vi "Network Address Lookup Table.vi"(7 "Action":T3, 8 "error in (no error)":errorcluster, 9 "Address":u8, 10 "Data":T2 {"Name" format="%.0x"}, 11 "Address LUT":T1) -> (0 "error out":errorcluster {"code" min=0 max=0}, 1 "Found?":bool, 2 "Data":T2 {"Name" format="%.0x"}, 3 "Address LUT out":T1, 4 "All Data":T2[](array[typedef]) {"Name" format="%.0x"})   [LabVIEW 2015, in "J1939 Addon Engine.lvlib"]
uses:
  J1939 Addon Engine.lvlib
  J1939 Multi Packet Frame/Types/Address Table Reference.ctl
  Shared/Types/Address Lookup Table Data.ctl
  J1939 Multi Packet Frame/Types/Address Lookup Table Action.ctl
  Shared/J1939 Addon Shared.lvlib
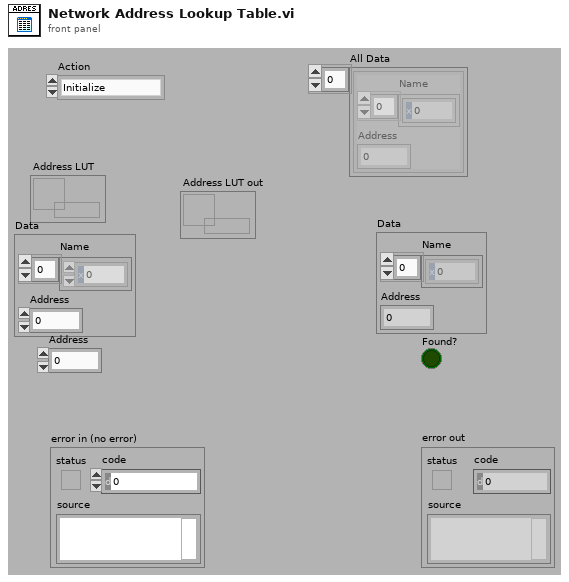
[diagram p1: front panel]
types:
  T1 = typedef "J1939 Addon Engine.lvlib/Address Table Reference.ctl" = refnum<data-value>
  T2 = typedef "J1939 Addon Shared.lvlib/Address Lookup Table Data.ctl" = cluster{"Name":u8[], "Address":u8}
  T3 = typedef "J1939 Addon Engine.lvlib/Address Lookup Table Action.ctl" = enum16{"Initialize", "Add", "Get", "Remove", "Get All"}
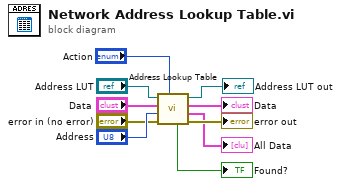
[diagram p0: block diagram]
diagram:
  n1 = call "Address Lookup Table.vi"("Action"="Action", "error in (no error)"="error in (no error)", "Address"="Address", "Data"="Data", "Address LUT"="Address LUT") -> ("error out"=→"error out":errorcluster, "All Data"=→"All Data":T2[], "Data"=→"Data":T2, "Address LUT out"=→"Address LUT out":T1, "Found?"=→"Found?":bool)  [unwired: 2 in]
